vi "Configure Channel Characteristics.vi"(5 "Enable Bandwidth Limit (F: Disable)":bool, 6 "Enable Vernier (F: Disable)":bool, 7 "Enable Invert (F: Disable)":bool, 8 "error in (no error)":errorcluster, 9 "Unit (0: Volt)":i32(ring) items=["Volt", "Ampere"], 10 "Channel Name (0: Channel 1)":i32(ring) items=["Channel 1", "Channel 2", "Channel 3", "Channel 4"], 11 "VISA resource name":refnum<visa-resource-name>) -> (0 "error out":errorcluster, 3 "VISA resource name out":refnum<visa-resource-name>)   [LabVIEW 2017, in "Agilent 2000 3000 X-Series.lvlib"]
doc: "Configures the common properties of the vertical subsystem of the oscilloscope for the specified channel. Call this VI for each channel you want to enable to acquire waveforms.\n\n<B>Note(s):</B>\nThe channel settings will not be applied if the channel is not enabled."
uses:
  Agilent 2000 3000 X-Series.lvlib
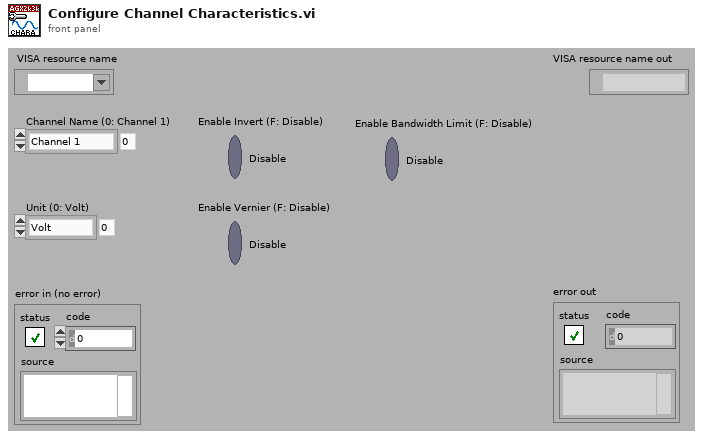
[diagram p1: front panel]
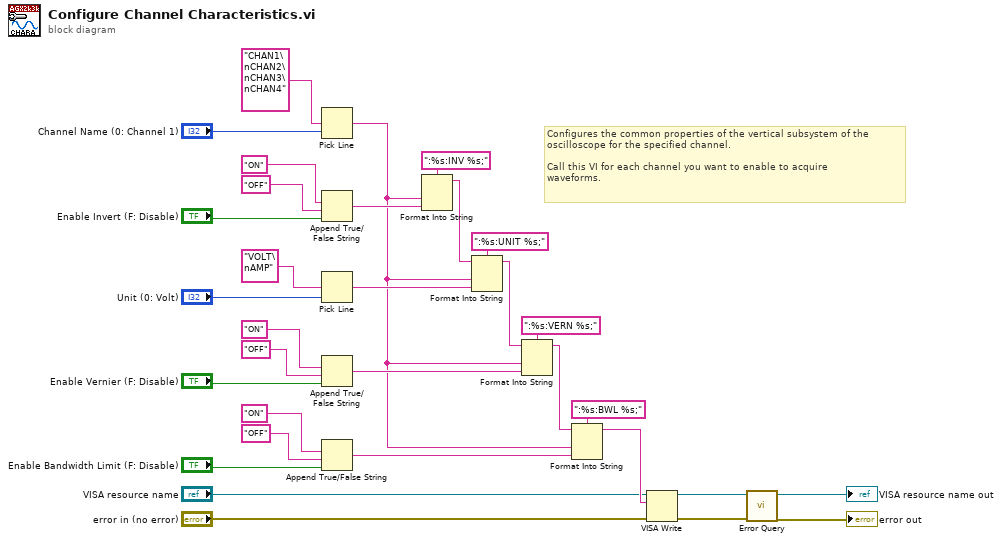
[diagram p0: block diagram]
diagram:
  # "Configures the common properties of the vertical subsystem of the \noscilloscope for the specified channel.  \n\nCall this VI for each channel you want to enable to acquire \nwaveforms."
  n1 = Pick Line(multi-line string="CHAN1\nCHAN2\nCHAN3\nCHAN4", line index="Channel Name (0: Channel 1)") -> (output string=w1:string)  [unwired: 1 out]
  n2 = Append True/False String(1:"Enable Invert (F: Disable)", 2:"OFF", 3:"ON") -> (0:w28:string)  [unwired: 1 out]
  n3 = Pick Line(multi-line string="VOLT\nAMP", line index="Unit (0: Volt)") -> (output string=w23:string)  [unwired: 1 out]
  n4 = Append True/False String(1:"Enable Vernier (F: Disable)", 2:"OFF", 3:"ON") -> (0:w17:string)  [unwired: 1 out]
  n5 = Append True/False String(1:"Enable Bandwidth Limit (F: Disable)", 2:"OFF", 3:"ON") -> (0:w11:string)  [unwired: 1 out]
  n6 = Format Into String(format string=":%s:INV %s;", w1, w28) -> (resulting string=w25:string)  [unwired: 2 in, 1 out]
  n7 = Format Into String(format string=":%s:UNIT %s;", initial string=w25, w1, w23) -> (resulting string=w19:string)  [unwired: 1 in, 1 out]
  n8 = Format Into String(format string=":%s:VERN %s;", initial string=w19, w1, w17) -> (resulting string=w13:string)  [unwired: 1 in, 1 out]
  n9 = Format Into String(format string=":%s:BWL %s;", initial string=w13, w1, w11) -> (resulting string=w10:string)  [unwired: 1 in, 1 out]
  n10 = VISA Write(VISA resource name="VISA resource name", write buffer=w10, error in (no error)="error in (no error)") -> (VISA resource name out=w7:refnum<visa-resource-name>, error out=w6:errorcluster)  [unwired: 1 out]
  n11 = call "Error Query.vi"("error in (no error)"=w6, "VISA resource name"=w7) -> ("error out"=→"error out":errorcluster, "VISA resource name out"=→"VISA resource name out":refnum<visa-resource-name>)  [unwired: 8 out]
